vi "Construct Stimulus Spot (SubVI).vi"(0 "DMD1X Array":dbl[][](array[numeric]), 1 "DMD1Y Array":dbl[][](array[numeric]), 2 "DMD2X Array":dbl[][](array[numeric]), 3 "DMD2Y Array":dbl[][](array[numeric]), 6 "Width":i32, 8 "Height":i32, 10 "Y":i32, 12 "X":i32) -> (14 "DMD1Y":i32, 15 "DMD1X":i32, 16 "DMD1 Array":u8[][](array[numeric]), 17 "DMD2Y":i32, 18 "DMD2X":i32, 19 "DMD2 Array":u8[][](array[numeric]))   [LabVIEW 2017]
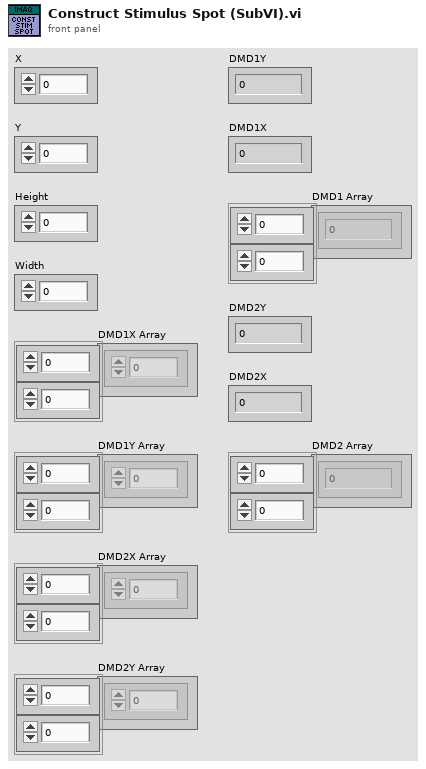
[diagram p1: front panel]
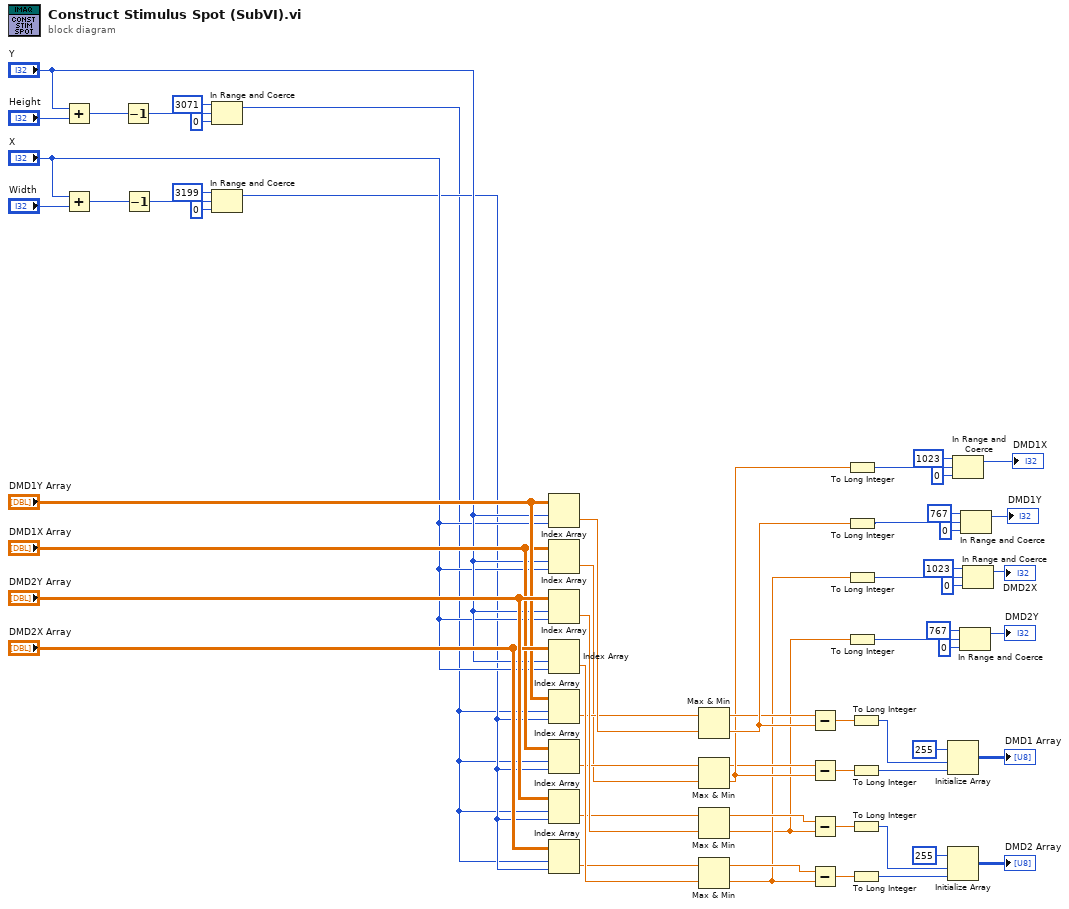
[diagram p0: block diagram]
diagram:
  n1 = Add(x="Y", y="Height") -> (x+y=w57:i32)
  n2 = Add(x="X", y="Width") -> (x+y=w58:i32)
  n3 = Decrement(x=w57) -> (x-1=w18:i32)
  n4 = Decrement(x=w58) -> (x-1=w20:i32)
  n5 = In Range and Coerce(upper limit=3071 ("x"), x=w18, lower limit=0) -> (coerced(x)=w23:i32)  [unwired: 1 out]
  n6 = In Range and Coerce(upper limit=3199 ("x"), x=w20, lower limit=0) -> (coerced(x)=w24:i32)  [unwired: 1 out]
  n7 = Index Array(array="DMD1Y Array", index (row)="Y", index (col)="X") -> (element=w44:dbl)
  n8 = Index Array(array="DMD1X Array", index (row)="Y", index (col)="X") -> (element=w35:dbl)
  n9 = Index Array(array="DMD2Y Array", index (row)="Y", index (col)="X") -> (element=w60:dbl)
  n10 = Index Array(array="DMD2X Array", index (row)="Y", index (col)="X") -> (element=w59:dbl)
  n11 = Index Array(array="DMD1Y Array", index (row)=w23, index (col)=w24) -> (element=w43:dbl)
  n12 = Index Array(array="DMD1X Array", index (row)=w23, index (col)=w24) -> (element=w42:dbl)
  n13 = Index Array(array="DMD2Y Array", index (row)=w23, index (col)=w24) -> (element=w53:dbl)
  n14 = Index Array(array="DMD2X Array", index (row)=w23, index (col)=w24) -> (element=w54:dbl)
  n15 = Max & Min(x=w43, y=w44) -> (max(x,y)=w48:dbl, min(x,y)=w49:dbl)
  n16 = Max & Min(x=w42, y=w35) -> (max(x,y)=w45:dbl, min(x,y)=w46:dbl)
  n17 = Max & Min(x=w53, y=w60) -> (max(x,y)=w51:dbl, min(x,y)=w21:dbl)
  n18 = Max & Min(x=w54, y=w59) -> (max(x,y)=w52:dbl, min(x,y)=w22:dbl)
  n19 = Subtract(x=w48, y=w49) -> (x-y=w50:dbl)
  n20 = Subtract(x=w45, y=w46) -> (x-y=w47:dbl)
  n21 = Subtract(x=w51, y=w21) -> (x-y=w62:dbl)
  n22 = Subtract(x=w52, y=w22) -> (x-y=w61:dbl)
  n23 = To Long Integer(number=w46) -> (32bit integer=w14:i32)
  n24 = To Long Integer(number=w49) -> (32bit integer=w10:i32)
  n25 = To Long Integer(number=w22) -> (32bit integer=w5:i32)
  n26 = To Long Integer(number=w21) -> (32bit integer=w1:i32)
  n27 = To Long Integer(number=w50) -> (32bit integer=w28:i32)
  n28 = To Long Integer(number=w47) -> (32bit integer=w29:i32)
  n29 = To Long Integer(number=w62) -> (32bit integer=w32:i32)
  n30 = To Long Integer(number=w61) -> (32bit integer=w33:i32)
  n31 = Initialize Array(u8 255 ("element"), w28, w29) -> (→"DMD1 Array":u8[][])
  n32 = Initialize Array(u8 255 ("element"), w32, w33) -> (→"DMD2 Array":u8[][])
  n33 = In Range and Coerce(upper limit=1023 ("x"), x=w14, lower limit=0) -> (coerced(x)=→"DMD1X":i32)  [unwired: 1 out]
  n34 = In Range and Coerce(upper limit=767 ("x"), x=w1, lower limit=0) -> (coerced(x)=→"DMD2Y":i32)  [unwired: 1 out]
  n35 = In Range and Coerce(upper limit=767 ("x"), x=w10, lower limit=0) -> (coerced(x)=→"DMD1Y":i32)  [unwired: 1 out]
  n36 = In Range and Coerce(upper limit=1023 ("x"), x=w5, lower limit=0) -> (coerced(x)=→"DMD2X":i32)  [unwired: 1 out]
